vi "Example Debug Code.vi"() -> ()   [LabVIEW 2021]
uses:
  <userlib>/_OpenG.lib/string/string.llb/Convert EOLs (String)__ogtk.vi
panel:
  in  "Input":string="46threevqs8114\nthreetwoonez1gtrd\n6ffxbtff\n769twotwo6rv9\ngjrcjrkvghthreegqqrg82qbct\nzkxjhgprtrlcfeight795five8\n99seven3vdcgvmvxtjtwodc5\nthree5eightthree3four3vtkkqrgxs\nfour863mrrnrsxrkone\nsevenntgvnrrqfvxh2ttnkgffour8fiveone\n49fbsfb\n3rbmlsksg\nztgszqjjsrtmgqx6572\n3bqnfxkdbonesixseven\nmfgx32ftpbhgngm7\nfzrpfhbfvj6dbxbtfs7twofksfbshrzkdeightwoqg\n2xcftwo\ncshmmltsml4fiveeightdn\neightthsix1\ntwo1gvfxcqnrfnbeightthreexznhbmmk\n3917sevenvxqxntcgxskh\nksctcnfxdsk96drlbjkthreesfqlvnpvfbcbmg\n8nvrmzfs46\n5dbgltmgg1xvtqfkdxsrxzltwo1pgqlqndlc\neight7four6rpbtmjzj5\n41seven\ngpmfhninexxgqr6\n15sixdrhxzcmqf\n8fivettgmcs..."
  out "Output":i64
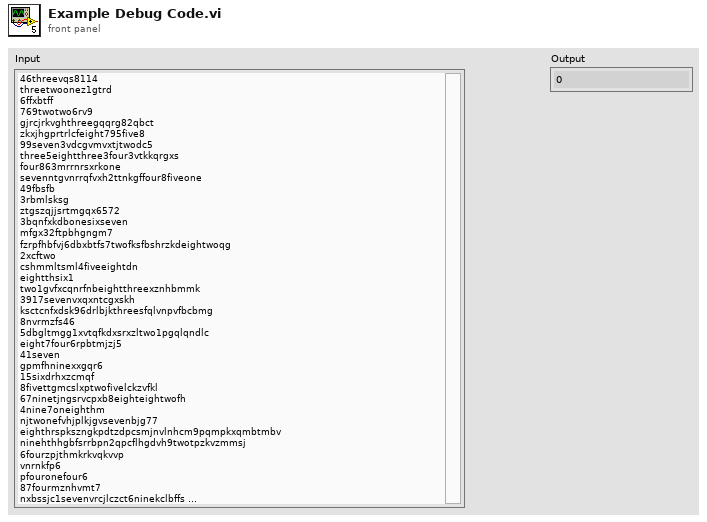
[diagram p1: front panel]
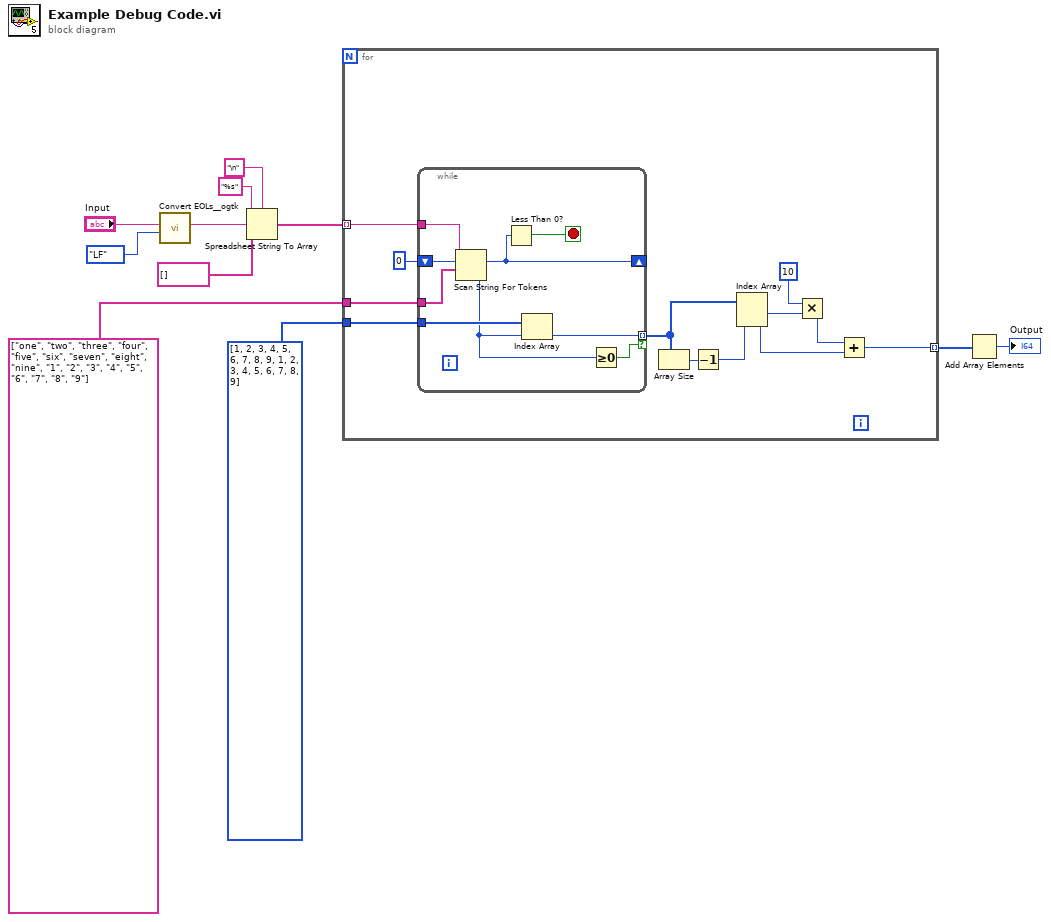
[diagram p0: block diagram]
diagram:
  n1 = call-poly <userlib>:"Convert EOLs__ogtk.vi"("Convert to:"=enum16{"CR", "LF", "CRLF"}."LF", "String in"="Input") -> ("String out"=w7:string)  [unwired: 9 in]
  n2 = Spreadsheet String To Array(delimiter (Tab)="\n", format string="%s", spreadsheet string=w7, array type (2D Dbl)=string[] []) -> (array=w5:string[])
  n3 = for {
    tunnel: w5 -> [w21] mode=indexing
    tunnel: [w16] -> w4 mode=indexing
    tunnel: string[] ["one", "two", "three", "four", "five", "six", "seven", "eight", "nine", "1", "2", "3", "4", "5", "6", "7", "8", "9"] -> [w23]
    tunnel: i64[] [1, 2, 3, 4, 5, 6, 7, 8, 9, 1, 2, 3, 4, 5, 6, 7, 8, 9] -> [w22]
    n4 = while {
      tunnel: w23 -> [w26]
      tunnel: w22 -> [w32]
      shift-right: [w30] -> _
      shift-left: 0 -> [w29]
      tunnel: [w28] -> w15 mode=indexing if=w24
      tunnel: w21 -> [w27]
      stop <- w31 stop-if-true
      n5 = Scan String For Tokens(7:w26, 8:w29, 9:w27) -> (0:w25:i32, 2:w30:i32)  [unwired: 3 in, 2 out]
      n6 = Less Than 0?(x=w30) -> (x < 0?=w31:bool)
      n7 = Index Array(array=w32, index=w25) -> (element=w28:i64)
      n8 = Greater Or Equal To 0?(x=w25) -> (x >= 0?=w24:bool)
    }
    n9 = Array Size(array=w15) -> (size(s)=w14:i32)
    n10 = Decrement(x=w14) -> (x-1=w13:i32)
    n11 = Index Array(array=w15, index #2=w13) -> (element #1=w19:i64, element #2=w12:i64)  [unwired: 1 in]
    n12 = Multiply(x=i64 10, y=w19) -> (x*y=w17:i64)
    n13 = Add(x=w17, y=w12) -> (x+y=w16:i64)
  }
  n14 = Add Array Elements(numeric array=w4) -> (sum=→"Output":i64)
